vi "Shutdown.vi"(8 "error in (no error)":errorcluster, 11 "Abstract Producer in":refnum<class "Abstract Producer.lvclass">) -> (0 "error out":errorcluster, 3 "Abstract Producer out":refnum<class "Abstract Producer.lvclass">)   [LabVIEW 2017, in "Messaging.lvlib" / "Abstract Producer.lvclass"]
uses:
  Abstract Producer.lvclass
  Abstract Producer.lvclass/Abstract Producer.ctl
  Consumer Information.ctl
  Message Queue/Abstract Message Queue/Abstract Message Queue.lvclass
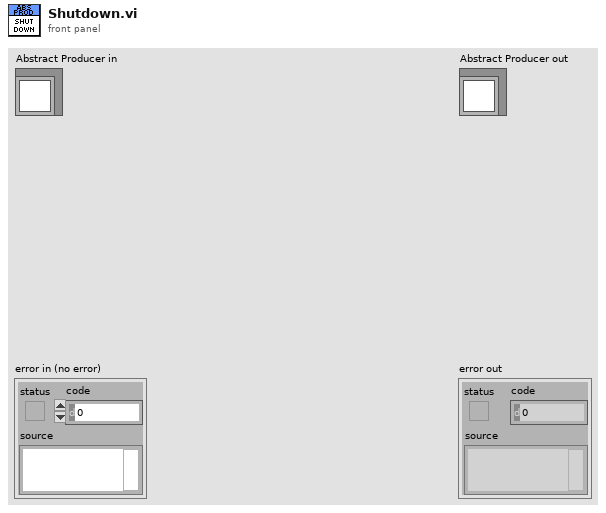
[diagram p1: front panel]
types:
  T1 = typedef "Messaging.lvlib/Abstract Producer.lvclass/Consumer Information.ctl" = cluster{"Name":string, "Request Queue":refnum<class "Abstract Message Queue.lvclass">, "Response Queue":refnum<class "Abstract Message Queue.lvclass">}
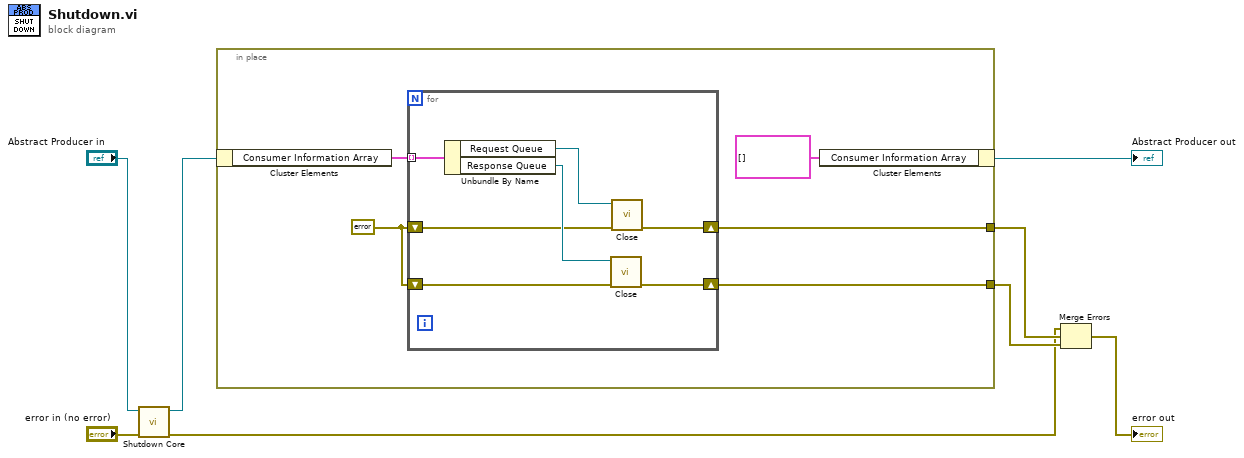
[diagram p0: block diagram]
diagram:
  n1 = call-dynamic "Shutdown Core.vi"("error in (no error)"="error in (no error)", "Abstract Producer in"="Abstract Producer in") -> ("error out"=w3:errorcluster, "Abstract Producer out"=w1:refnum<class "Abstract Producer.lvclass">)  [unwired: 8 in]
  n2 = in-place {
    in-place-border: [w10] -> w6
    in-place-border: [w9] -> w5
    w11 = errorcluster {"status"=FALSE, "code"=0, "source"=""} ("error out")
    n3 = in-place-cluster #1(w1) -> ("Consumer Information Array"=w12:T1[])
    n4 = for {
      tunnel: w12 -> [w20] mode=indexing
      shift-right: [w16] -> w9
      shift-left: w11 -> [w15]
      shift-right: [w17] -> w10
      shift-left: w11 -> [w14]
      n5 = Unbundle By Name(w20) -> ("Request Queue"=w19:refnum<class "Abstract Message Queue.lvclass">, "Response Queue"=w18:refnum<class "Abstract Message Queue.lvclass">)
      n6 = call-dynamic "Close.vi"("error in (no error)"=w14, "Abstract Message Queue in"=w18) -> ("error out"=w17:errorcluster)  [unwired: 8 in, 1 out]
      n7 = call-dynamic "Close.vi"("error in (no error)"=w15, "Abstract Message Queue in"=w19) -> ("error out"=w16:errorcluster)  [unwired: 8 in, 1 out]
    }
    n8 = in-place-cluster #1("Consumer Information Array"=T1[] []) -> (→"Abstract Producer out":refnum<class "Abstract Producer.lvclass">)
  }
  n9 = Merge Errors(w3, w5, w6) -> (→"error out":errorcluster)
